vi "testSendEvent.vi"(8 "error in (no error)":errorcluster) -> (0 "error out":errorcluster)   [LabVIEW 2018]
doc: "Test the checkCallback.vi"
uses:
  src/TcpServer/TcpServer.lvclass
  <vilib>/addons/_JKI Toolkits/Caraya/classes/Assert/Assert Equal Value_Variant.vi
  <vilib>/addons/_JKI Toolkits/Caraya/classes/Test/Test.lvclass
  <vilib>/addons/_JKI Toolkits/Caraya/classes/Assert/Assert.lvclass
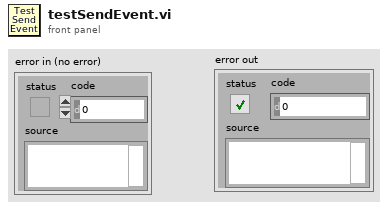
[diagram p1: front panel]
types:
  T1 = typedef "userEventsTypeDef.ctl" = cluster{"TcpServer":refnum<user-event>, "Command":refnum<user-event>, "CmdStatus":refnum<user-event>, "Event":refnum<user-event>, "Telemetry":refnum<user-event>}
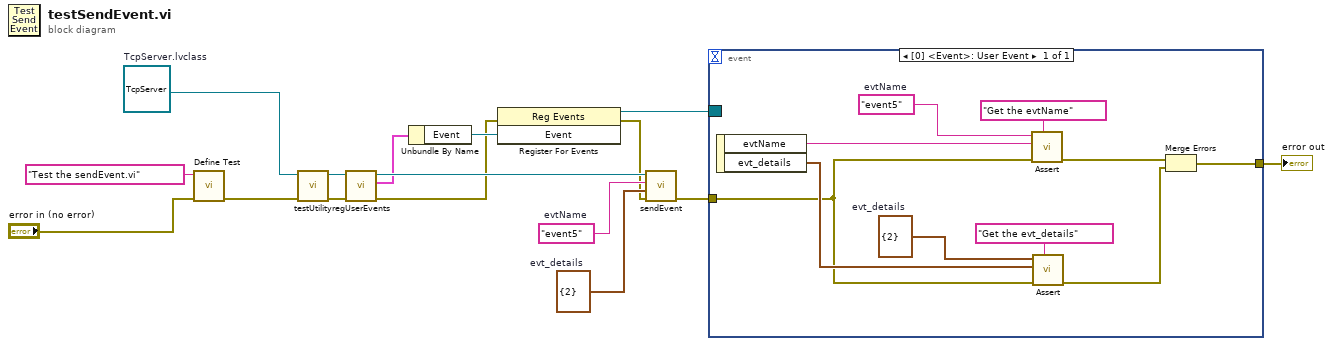
[diagram p0: block diagram]
diagram:
  w10 = cluster{"state":i32} {"state"=2}  # evt_details
  w11 = "event5"  # evtName
  w13 = refnum<class "TcpServer.lvclass"> refnum  # TcpServer.lvclass
  n1 = call <vilib>:"Define Test.vi"("error in (no error)"="error in (no error)", "Label (VI Title)"="Test the sendEvent.vi") -> ("error out"=w15:errorcluster)  [unwired: 9 in]
  n2 = call "testUtility.vi"("error in (no error)"=w15, "TcpServer.lvclass"=w13) -> ("error out"=w12:errorcluster, "tcpServer out"=w9:refnum<class "TcpServer.lvclass">)  [unwired: 8 in]
  n3 = call "regUserEvents.vi"("error in (no error)"=w12, "tcpServer in"=w9) -> ("error out"=w3:errorcluster, "UserEvents"=w7:T1, "tcpServer out"=w8:refnum<class "TcpServer.lvclass">)  [unwired: 7 in]
  n4 = Unbundle By Name(w7) -> ("Event"=w6:refnum<user-event>)
  n5 = register-events(error in=w3, w6) -> (reference out=w5:refnum<event-registration>, error out=w2:errorcluster)  [unwired: 1 in]
  n6 = call "sendEvent.vi"("error in (no error)"=w2, "evt_details"=w10, "evtName"=w11, "TcpServer in"=w8) -> ("error out"=w1:errorcluster)  [unwired: 6 in, 1 out]
  n7 = event shown="[0] <Event>: User Event" {
    selector: w5 -> [_]
    dyn-events: _ -> [_]
    timeout: _ -> [_]
    tunnel: w1 -> [w17]
    tunnel: [w19] -> w4
    event User Event {
      w21 = "event5"  # evtName
      w23 = cluster{"state":i32} {"state"=2}  # evt_details
      n8 = event-data() -> ("evtName"=w18:string, "evt_details"=w20:cluster{"state":i32})  [unwired: 1 in]
      n9 = call-poly <vilib>:"Assert.vi"("Label"="Get the evtName", "error in (no error)"=w17, "Y"=w18, "X"=w21) -> ("error out"=w25:errorcluster)  [unwired: 7 in]
      n10 = call-poly <vilib>:"Assert.vi"("Label"="Get the evt_details", "error in (no error)"=w17, "Y"=w20, "X"=w23) -> ("error out"=w26:errorcluster)  [unwired: 7 in]
      n11 = Merge Errors(w25, w26) -> (w19:errorcluster)
    }
  }
  "error out" <- w4
